vi "7-29-19 300k Decreasing extrapolation.vi"() -> ()   [LabVIEW 2016]
uses:
  <vilib>/Analysis/baseanly.llb/Mean (DBL).vi
  <userlib>/Levylab/LV to ITX/LVtoITX.lvclass
  <vilib>/Analysis/NI_AALPro.lvlib
  <vilib>/Analysis/NI_AALBase.lvlib
panel:
  out "dG/dt/G vs Temp":cluster{dbl[], dbl[]}[](graph)
  out "dG/dt vs Temp":cluster{dbl[], dbl[]}[](graph)
  out "dG/dt Vs Temp Normalized":cluster{"Data":dbl[], "Data":dbl[]}[](graph)
  out "G Vs Time Fitted":cluster{"Data":dbl[], "Data":dbl[]}[](graph)
  out "G Vs Time 2":cluster{dbl[], dbl[]}[](graph)
  out "G Vs Time":cluster{"Data":dbl[], "Data":dbl[]}[](graph)
  in  "parameter bounds":T1={"amp min"=-inf, "amp max"=inf, "damping min"=-inf, "damping max"=inf, "offset min"=-inf, "offset max"=inf}
  in  "Path":path=path "G:/My Drive/Data/7-30 Decreasing SA03083.dat"
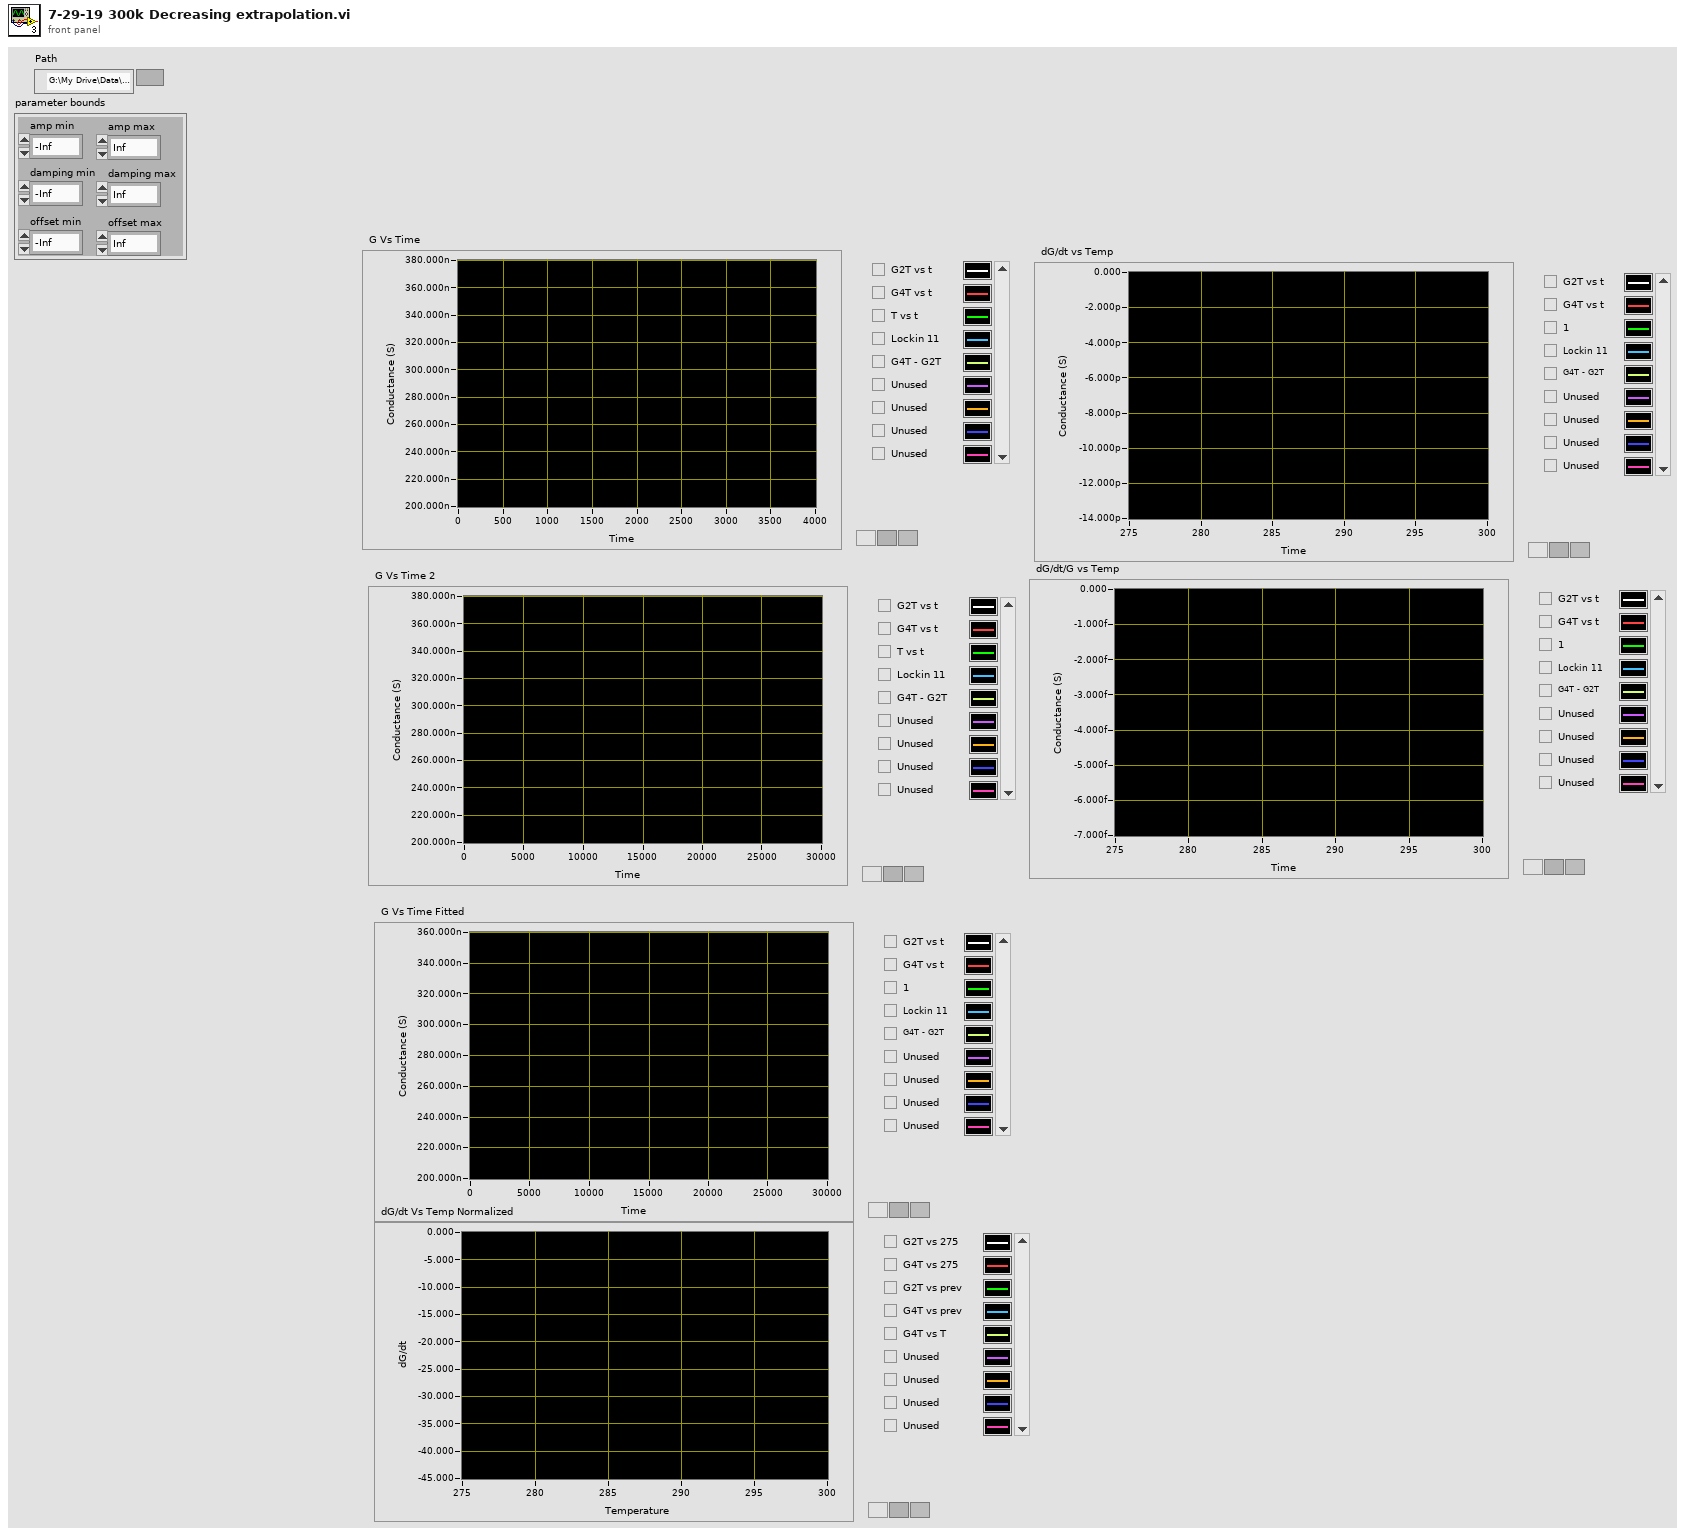
[diagram p1: front panel]
types:
  T1 = cluster{"amp min":dbl, "amp max":dbl, "damping min":dbl, "damping max":dbl, "offset min":dbl, "offset max":dbl}
  T2 = cluster{"slope min":dbl, "slope max":dbl, "intercept min":dbl, "intercept max":dbl}
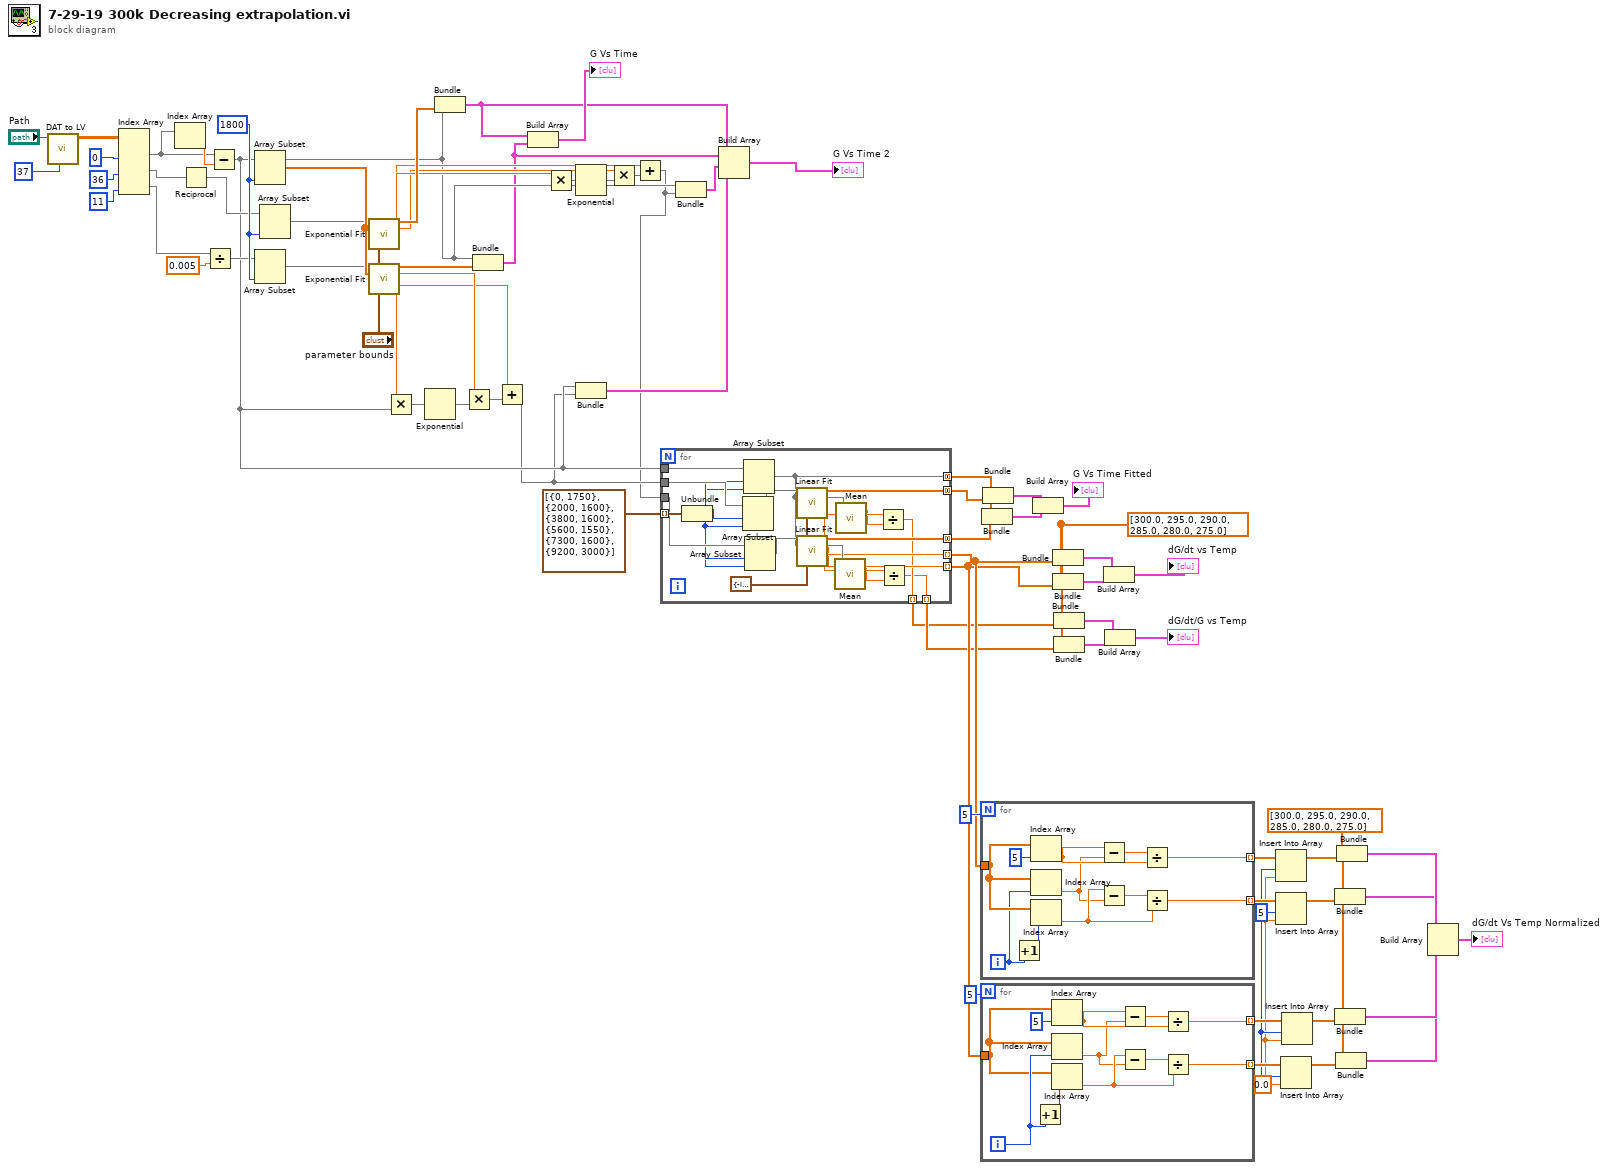
[diagram p0: block diagram]
diagram:
  w3 = dbl[] [300.0, 295.0, 290.0, 285.0, 280.0, 275.0]
  w22 = dbl[] [300.0, 295.0, 290.0, 285.0, 280.0, 275.0]
  w27 = 0.0 ("new element/subarray")
  w28 = 5 ("index")
  w68 = 1800
  n1 = call <userlib>:"DAT to LV.vi"("header length"=37, "File Path"="Path") -> ("Data"=w75:dbl[][])  [unwired: 6 in, 3 out]
  n2 = Index Array(array=w75, index (col) #1=0 ("disabled index (col)"), index (col) #2=36 ("index (col)"), index (col) #3=11 ("index (col)")) -> (element #1=w51:dbl[], element #2=w69:dbl[], element #3=w71:dbl[])  [unwired: 3 in]
  n3 = Index Array(array=w51) -> (element=w58:dbl)  [unwired: 1 in]
  n4 = Reciprocal(x=w69) -> (1/x=w63:dbl[])
  n5 = Divide(x=w71, y=0.005) -> (x/y=w62:dbl[])
  n6 = Subtract(x=w51, y=w58) -> (x-y=w16:dbl[])
  n7 = Array Subset(array=w16, length=w68) -> (w61:dbl[])  [unwired: 1 in]
  n8 = Array Subset(array=w62, length=w68) -> (w60:dbl[])  [unwired: 1 in]
  n9 = Array Subset(array=w63, length=w68) -> (w59:dbl[])  [unwired: 1 in]
  n10 = call <vilib>:"Exponential Fit.vi"("Y"=w59, "X"=w61, "parameter bounds"="parameter bounds") -> ("Best Exponential Fit"=w67:dbl[], "amplitude"=w46:dbl, "damping"=w47:dbl, "offset"=w45:dbl)  [unwired: 7 in, 2 out]
  n11 = call <vilib>:"Exponential Fit.vi"("Y"=w60, "X"=w61, "parameter bounds"="parameter bounds") -> ("Best Exponential Fit"=w66:dbl[], "amplitude"=w56:dbl, "damping"=w57:dbl, "offset"=w52:dbl)  [unwired: 7 in, 2 out]
  n12 = Multiply(x=w57, y=w16) -> (x*y=w55:dbl[])
  n13 = Exponential(1:w55) -> (0:w54:dbl[])
  n14 = Bundle(w16, "Best Exponential Fit"=w67) -> (w8:cluster{dbl[], "Best Exponential Fit":dbl[]})  [unwired: 1 in]
  n15 = Multiply(x=w56, y=w54) -> (x*y=w53:dbl[])
  n16 = Bundle(w16, "Best Exponential Fit"=w66) -> (w7:cluster{dbl[], "Best Exponential Fit":dbl[]})  [unwired: 1 in]
  n17 = Add(x=w52, y=w53) -> (x+y=w15:dbl[])
  n18 = Build Array(w8, w7) -> (→"G Vs Time":cluster{dbl[], "Best Exponential Fit":dbl[]}[])
  n19 = Multiply(x=w47, y=w16) -> (x*y=w48:dbl[])
  n20 = Exponential(1:w48) -> (0:w49:dbl[])
  n21 = Bundle(w16, w15) -> (w43:cluster{dbl[], dbl[]})  [unwired: 1 in]
  n22 = Multiply(x=w46, y=w49) -> (x*y=w50:dbl[])
  n23 = Add(x=w45, y=w50) -> (x+y=w14:dbl[])
  n24 = for {
    tunnel: cluster{"Index":i32, "Length":i32}[] [{"Index"=0, "Length"=1750}, {"Index"=2000, "Length"=1600}, {"Index"=3800, "Length"=1600}, {"Index"=5600, "Length"=1550}, {"Index"=7300, "Length"=1600}, {"Index"=9200, "Length"=3000}] -> [w95] mode=indexing
    tunnel: w16 -> [w94]
    tunnel: w15 -> [w93]
    tunnel: w14 -> [w92]
    tunnel: [w88] -> w39 mode=concatenating
    tunnel: [w87] -> w38 mode=concatenating
    tunnel: [w83] -> w13 mode=indexing
    tunnel: [w82] -> w9 mode=indexing
    tunnel: [w84] -> w40 mode=concatenating
    tunnel: [w79] -> w4 mode=indexing
    tunnel: [w78] -> w5 mode=indexing
    w89 = T2 {"slope min"=-inf, "slope max"=inf, "intercept min"=-inf, "intercept max"=inf} ("parameter bounds")
    n25 = Unbundle(w95) -> ("Index"=w91:i32, "Length"=w90:i32)
    n26 = Array Subset(array=w93, index=w91, length=w90) -> (w86:dbl[])
    n27 = Array Subset(array=w94, index=w91, length=w90) -> (w84:dbl[])
    n28 = Array Subset(array=w92, index=w91, length=w90) -> (w85:dbl[])
    n29 = call <vilib>:"Linear Fit.vi"("Y"=w86, "X"=w84, "parameter bounds"=w89) -> ("Best Linear Fit"=w88:dbl[], "slope"=w83:dbl)  [unwired: 8 in, 3 out]
    n30 = call <vilib>:"Linear Fit.vi"("Y"=w85, "X"=w84, "parameter bounds"=w89) -> ("Best Linear Fit"=w87:dbl[], "slope"=w82:dbl)  [unwired: 8 in, 3 out]
    n31 = call-poly <vilib>:"Mean.vi"("X"=w84) -> ("mean"=w81:dbl)  [unwired: 1 out]
    n32 = call-poly <vilib>:"Mean.vi"("X"=w84) -> ("mean"=w80:dbl)  [unwired: 1 out]
    n33 = Divide(x=w83, y=w80) -> (x/y=w79:dbl)
    n34 = Divide(x=w82, y=w81) -> (x/y=w78:dbl)
  }
  n35 = Bundle(w16, w14) -> (w44:cluster{dbl[], dbl[]})  [unwired: 1 in]
  n36 = Build Array(w8, w7, w44, w43) -> (→"G Vs Time 2":cluster{dbl[], "Best Exponential Fit":dbl[]}[])
  n37 = for {
    N: 5 -> [_]
    tunnel: w13 -> [w106]
    tunnel: [w100] -> w32 mode=indexing
    tunnel: [w99] -> w31 mode=indexing
    i -> [w104]
    n38 = Increment(x=w104) -> (x+1=w105:i32)
    n39 = Index Array(array=w106, index=5) -> (element=w98:dbl)
    n40 = Index Array(array=w106, index=w104) -> (element=w96:dbl)
    n41 = Index Array(array=w106, index=w105) -> (element=w97:dbl)
    n42 = Subtract(x=w98, y=w96) -> (x-y=w102:dbl)
    n43 = Subtract(x=w97, y=w96) -> (x-y=w101:dbl)
    n44 = Divide(x=w102, y=w98) -> (x/y=w100:dbl)
    n45 = Divide(x=w101, y=w97) -> (x/y=w99:dbl)
  }
  n46 = for {
    N: 5 -> [_]
    tunnel: w9 -> [w112]
    tunnel: [w111] -> w30 mode=indexing
    tunnel: [w110] -> w29 mode=indexing
    i -> [w113]
    n47 = Increment(x=w113) -> (x+1=w114:i32)
    n48 = Index Array(array=w112, index=5) -> (element=w109:dbl)
    n49 = Index Array(array=w112, index=w113) -> (element=w107:dbl)
    n50 = Index Array(array=w112, index=w114) -> (element=w108:dbl)
    n51 = Subtract(x=w109, y=w107) -> (x-y=w116:dbl)
    n52 = Subtract(x=w108, y=w107) -> (x-y=w117:dbl)
    n53 = Divide(x=w116, y=w109) -> (x/y=w111:dbl)
    n54 = Divide(x=w117, y=w108) -> (x/y=w110:dbl)
  }
  n55 = Bundle(w40, "Best Linear Fit"=w38) -> (w37:cluster{dbl[], "Best Linear Fit":dbl[]})  [unwired: 1 in]
  n56 = Bundle(w40, "Best Linear Fit"=w39) -> (w36:cluster{dbl[], "Best Linear Fit":dbl[]})  [unwired: 1 in]
  n57 = Build Array(w36, w37) -> (→"G Vs Time Fitted":cluster{dbl[], "Best Linear Fit":dbl[]}[])
  n58 = Bundle(w3, w13) -> (w12:cluster{dbl[], dbl[]})  [unwired: 1 in]
  n59 = Bundle(w3, w9) -> (w11:cluster{dbl[], dbl[]})  [unwired: 1 in]
  n60 = Bundle(w3, w4) -> (w2:cluster{dbl[], dbl[]})  [unwired: 1 in]
  n61 = Bundle(w3, w5) -> (w6:cluster{dbl[], dbl[]})  [unwired: 1 in]
  n62 = Build Array(w12, w11) -> (→"dG/dt vs Temp":cluster{dbl[], dbl[]}[])
  n63 = Build Array(w2, w6) -> (→"dG/dt/G vs Temp":cluster{dbl[], dbl[]}[])
  n64 = Insert Into Array(array=w32, index=w28, new element=w27) -> (w24:dbl[])
  n65 = Insert Into Array(array=w31, index=w28, new element=w27) -> (w23:dbl[])
  n66 = Insert Into Array(array=w29, index=w28, new element=w27) -> (w25:dbl[])
  n67 = Insert Into Array(array=w30, index=w28, new element=w27) -> (w26:dbl[])
  n68 = Bundle(w22, w23) -> (w19:cluster{dbl[], dbl[]})  [unwired: 1 in]
  n69 = Bundle(w22, w26) -> (w21:cluster{dbl[], dbl[]})  [unwired: 1 in]
  n70 = Bundle(w22, w25) -> (w18:cluster{dbl[], dbl[]})  [unwired: 1 in]
  n71 = Bundle(w22, w24) -> (w20:cluster{dbl[], dbl[]})  [unwired: 1 in]
  n72 = Build Array(w20, w21, w19, w18) -> (→"dG/dt Vs Temp Normalized":cluster{dbl[], dbl[]}[])
